vi "Read ADC.vi"(8 "error in (no error)":errorcluster, 11 "ADS1115 in":refnum<class "Grove An In ADS1115.lvclass">) -> (0 "error out":errorcluster, 2 "Data Out":dbl, 3 "ADS1115 out":refnum<class "Grove An In ADS1115.lvclass">)   [LabVIEW 2020, in "CTI-Peripheral.lvlib" / "Grove An In ADS1115.lvclass"]
uses:
  Grove An In ADS1115.lvclass
  Grove An In ADS1115.lvclass/Grove An In ADS1115.ctl
  CTI/I2C Connection/I2C Connection.lvclass/I2C Connection.ctl
  CTI/Session/I2C Write Data.vi
  CTI/Session/I2C Read Data.vi
  CTI/I2C Connection/I2C Connection.lvclass
panel:
  out "Data":string
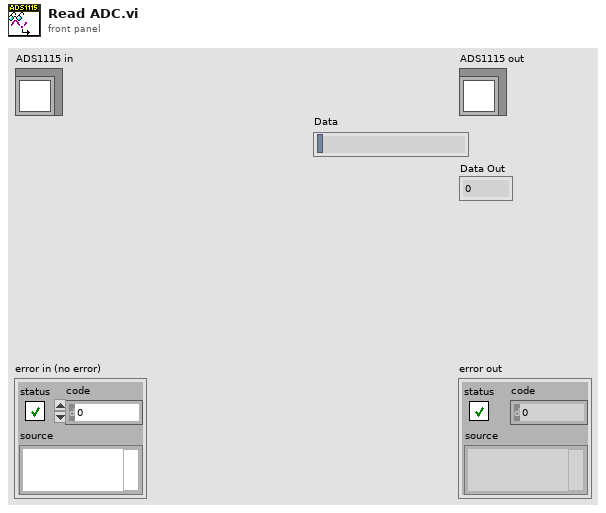
[diagram p1: front panel]
types:
  T1 = typedef "CTI-Peripheral.lvlib/Grove An In ADS1115.lvclass/ConfigData.ctl" = cluster{"Mode":T2, "MUX":T3, "Data Rate":T4, "PGA":T5}
  T2 = typedef "CTI-Peripheral.lvlib/Grove An In ADS1115.lvclass/ADS1115Mode.ctl" = enum16{"Continuous", "Single-Shot"}
  T3 = typedef "CTI-Peripheral.lvlib/Grove An In ADS1115.lvclass/ADS1115Mux.ctl" = enum16{"Single AI0 - GND", "Single AI1 - GND", "Single AI2 - GND", "Single AI3 - GND"}
  T4 = typedef "CTI-Peripheral.lvlib/Grove An In ADS1115.lvclass/ADS1115DataRate.ctl" = enum16{"8 SPS", "16 SPS", "32 SPS", "64 SPS", "128 SPS", "250 SPS", "475 SPS", "860 SPS"}
  T5 = typedef "CTI-Peripheral.lvlib/Grove An In ADS1115.lvclass/ADS1115PGA.ctl" = enum16{"FS = ±6.144V", "FS = ±4.096V", "FS = ±2.048V", "FS = ±1.024V", "FS = ±0.512V", "FS = ±0.256V"}
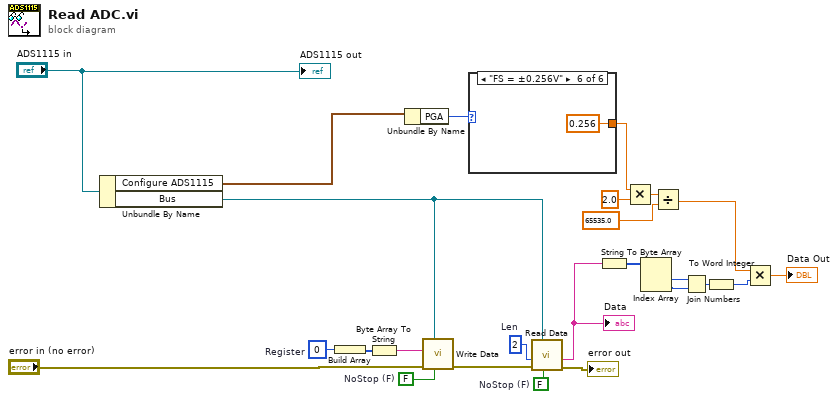
[diagram p0: block diagram]
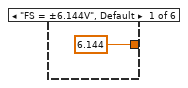
[diagram p2: hidden frame]
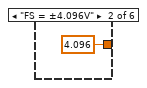
[diagram p3: hidden frame]
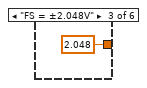
[diagram p4: hidden frame]
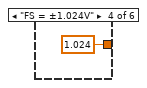
[diagram p5: hidden frame]
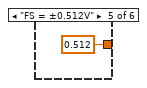
[diagram p6: hidden frame]
diagram:
  w12 = u8 0  # Register
  w21 = FALSE  # NoStop (F)
  w22 = u8 2  # Len
  w23 = FALSE  # NoStop (F)
  n1 = Unbundle By Name("ADS1115 in") -> ("Configure ADS1115"=w5:T1, "Bus"=w20:refnum<class "I2C Connection.lvclass">)
  n2 = Build Array(w12) -> (w13:u8[])
  n3 = Byte Array To String(unsigned byte array=w13) -> (string=w8:string)
  n4 = Unbundle By Name(w5) -> ("PGA"=w2:T5)
  n5 = call "Write Data.vi"("NoStop (F)"=w23, "I2C Connection"=w20, "error in (no error)"="error in (no error)", "Data"=w8) -> ("error out"=w19:errorcluster)  [unwired: 7 in]
  n6 = case shown="\"FS = ±0.256V\"" w2 {
    tunnel: [6.144 ("Waveform Chart") 4.096 ("Waveform Chart") 2.048 ("Waveform Chart") 1.024 ("Waveform Chart") 0.512 ("Waveform Chart") 0.256 ("Waveform Chart")] -> w1
    frame "FS = ±6.144V", Default {
    }
    frame "FS = ±4.096V" {
    }
    frame "FS = ±2.048V" {
    }
    frame "FS = ±1.024V" {
    }
    frame "FS = ±0.512V" {
    }
    frame "FS = ±0.256V" {
    }
  }
  n7 = call "Read Data.vi"("NoStop (F)"=w21, "I2C Connection"=w20, "error in (no error)"=w19, "Len"=w22) -> ("error out"=→"error out":errorcluster, "Data"=w7:string)  [unwired: 6 in]
  "Data" <- w7
  n8 = String To Byte Array(string=w7) -> (unsigned byte array=w17:u8[])
  n9 = Multiply(x=w1, y=2.0) -> (x*y=w11:dbl)
  n10 = Index Array(array=w17) -> (element #1=w16:u8, element #2=w15:u8)  [unwired: 2 in]
  n11 = Divide(x=w11, y=65535.0) -> (x/y=w3:dbl)
  n12 = Join Numbers(hi=w16, lo=w15) -> ((hi.lo)=w14:u16)
  n13 = To Word Integer(number=w14) -> (16bit integer=w4:i16)
  n14 = Multiply(x=w3, y=w4) -> (x*y=→"Data Out":dbl)
  "ADS1115 out" <- "ADS1115 in"
